vi "Home.vi"(8 "error in":errorcluster, 11 "Axis in":refnum<class "Axis.lvclass">) -> (0 "error out":errorcluster, 2 "Success?":bool, 3 "Axis out":refnum<class "Axis.lvclass">)   [LabVIEW 2018, in "Axis.lvlib" / "Axis.lvclass"]
uses:
  Axis.lvclass
  Custom Controls/Command.ctl
  Axis.lvlib
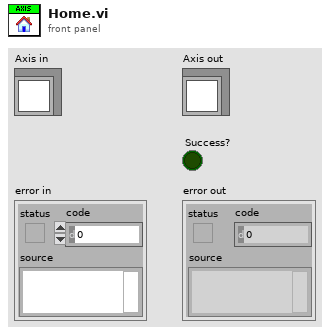
[diagram p1: front panel]
types:
  T1 = typedef "Axis.lvlib/Command.ctl" = enum16{"None", "Home", "Renumber", "Move Absolute", "Move Relative", "Stop", "Set Run Speed", "Set Acceleration", "Set Run Current", "Set Home Offset", "Set Home Speed", "Query Current Position", "Load Defaults", "Query Status", "Lock Controls", "Unlock Controls", "Set Jog Step Size", "Set Jog Acceleration", "Set Jog Speed", "Query Homed Status", "Query Moving Status", "Reset", "Set Max Position", "Set Min Position"}
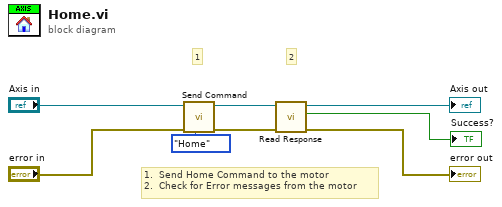
[diagram p0: block diagram]
diagram:
  # "1.  Send Home Command to the motor\n2.  Check for Error messages from the motor"
  # "2"
  # "1"
  n1 = call-dynamic "Send Command.vi"("Command"=Command."Home", "error in"="error in", "Axis in"="Axis in") -> ("error out"=w5:errorcluster, "Axis out"=w6:refnum<class "Axis.lvclass">)  [unwired: 7 in]
  n2 = call-dynamic "Read Response.vi"("error in"=w5, "Axis in"=w6) -> ("error out"=→"error out":errorcluster, "Success?"=→"Success?":bool, "Axis out"=→"Axis out":refnum<class "Axis.lvclass">)  [unwired: 7 in]
